vi "test Write Configuration File.vi"(8 "error in (no error)":errorcluster, 11 "TestCase in":refnum<class "Configuration Tests.lvclass">) -> (0 "error out":errorcluster, 3 "TestCase out":refnum<class "Configuration Tests.lvclass">)   [LabVIEW 2017, in "Configuration Tests.lvclass"]
uses:
  Configuration Tests.lvclass
  Configuration/Public/Controls/DSF Engine Framework Configuration.ctl
  Configuration/Public/Controls/DSF Engine Plugin Configuration.ctl
  Configuration/Public/Controls/DSF Timing Info.ctl
  Configuration/Public/Controls/DSF Engine Transfer Group Configuration.ctl
  Configuration/Public/Controls/DSF Direction.ctl
  Configuration/Public/Controls/DSF Engine Transfer Configuration.ctl
  Configuration/Public/Controls/DSF Byte Order.ctl
  Configuration/Public/Controls/DSF Engine Channel Configuration.ctl
  Configuration/Public/Controls/DSF Data Type.ctl
  Configuration/Public/Controls/DSF Settings Info.ctl
  Configuration/Public/Controls/DSF Plugin Info.ctl
  Configuration/Public/Controls/DSF Group Info.ctl
  Configuration/Public/Controls/DSF Transfer Info.ctl
  Configuration/Public/Controls/DSF Channel Info.ctl
  Configuration/Public/Write Item/Write Settings.vi
  Configuration/Public/Write Item/Write Channel.vi
  Configuration/Public/Write Item/Write Transfer.vi
  Configuration/Public/Write Item/Write Group.vi
  Configuration/Public/Write Item/Write Plugin.vi
  <vilib>/addons/_JKI Toolkits/VI Tester/TestCase.llb/TestCase.lvclass
  Configuration/Configuration Session.lvclass
  DSF Core.lvlib
  C:/Program Files (x86)/National Instruments/LabVIEW 2017/vi.lib/addons/_JKI Toolkits/VI Tester/TestCase.llb/TestCase.lvclass
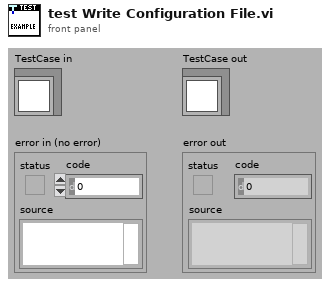
[diagram p1: front panel]
types:
  T1 = typedef "DSF Core.lvlib/DSF Settings Info.ctl" = cluster{"key":string, "value":string}[]
  T2 = typedef "DSF Core.lvlib/DSF Plugin Info.ctl" = cluster{"type":string, "timing":T3, "group ids":string[], "settings id":string, "thread count":i32}
  T3 = typedef "DSF Core.lvlib/DSF Timing Info.ctl" = cluster{"priority":u64, "decimation":u64, "offset":u64}
  T4 = typedef "DSF Core.lvlib/DSF Group Info.ctl" = cluster{"direction":T5, "timing":T3, "transfer ids":string[], "settings id":string}
  T5 = typedef "DSF Core.lvlib/DSF Direction.ctl" = enum8{"Tx", "Rx"}
  T6 = typedef "DSF Core.lvlib/DSF Transfer Info.ctl" = cluster{"byte order":T7, "channel ids":string[], "settings id":string}
  T7 = typedef "DSF Core.lvlib/DSF Byte Order.ctl" = enum8{"big-endian", "little-endian"}
  T8 = typedef "DSF Core.lvlib/DSF Channel Info.ctl" = cluster{"count":u64, "buffer offset":u64, "data type":T9, "settings id":string}
  T9 = typedef "DSF Core.lvlib/DSF Data Type.ctl" = enum8{"Bool", "SGL", "DBL", "I8", "I16", "I32", "I64", "U8", "U16", "U32", "U64"}
  T10 = typedef "DSF Core.lvlib/DSF Engine Framework Configuration.ctl" = cluster{"Plugins":T11[]}
  T11 = typedef "DSF Core.lvlib/DSF Engine Plugin Configuration.ctl" = cluster{"name":string, "class":string, "cycle timing":T3, "Transfer Groups":T12[], "settings":T1, "thread count":i32}
  T12 = typedef "DSF Core.lvlib/DSF Engine Transfer Group Configuration.ctl" = cluster{"name":string, "direction":T5, "cycle timing":T3, "Transfers":T13[], "settings":T1}
  T13 = typedef "DSF Core.lvlib/DSF Engine Transfer Configuration.ctl" = cluster{"name":string, "byte order":T7, "channel configurations":T14[], "settings":T1}
  T14 = typedef "DSF Core.lvlib/DSF Engine Channel Configuration.ctl" = cluster{"engine offset":u64, "name":string, "data type":T9, "count":u64, "buffer offset":u64}
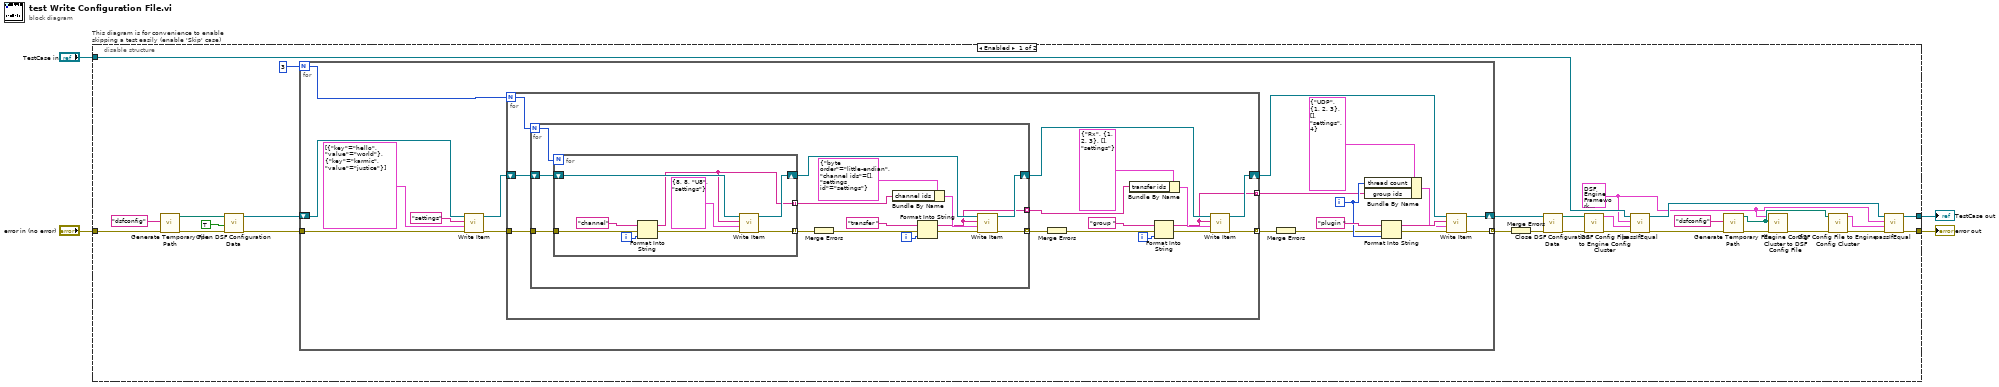
[diagram p0: block diagram]
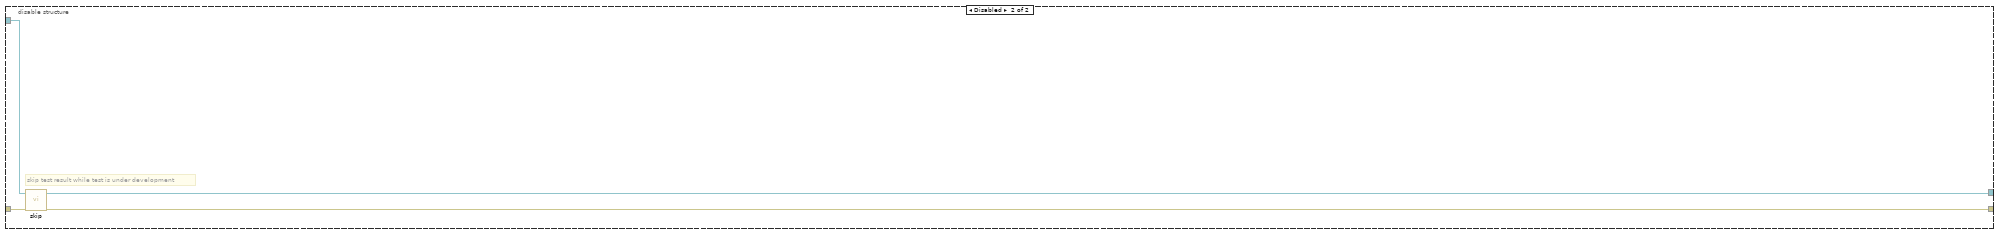
[diagram p2: hidden frame]
diagram:
  n1 = disable-structure "This diagram is for convenience to enable skipping a test easily (enable 'Skip' case)" shown="Enabled" {
    disable-tunnel: "TestCase in" -> [w18 w93]
    disable-tunnel: [w10 w91] -> w1
    disable-tunnel: [w12 w92] -> w3
    disable-tunnel: "error in (no error)" -> [w31 w90]
    frame Enabled {
      w5 = T10 {"Plugins"=[{"name"="plugin 0", "class"="UDP", "cycle timing"={"priority"=1, "decimation"=2, "offset"=3}, "Transfer Groups"=[{"name"="group 0", "direction"=enum."Rx", "cycle timing"={"priority"=1, "decimation"=2, "offset"=3}, "Transfers"=[{"name"="transfer 0", "byte order"=enum."little-endian", "channel configurations"=[{"engine offset"=0, "name"="channel0", "data type"=enum."U8", "count"=8, "buffer offset"=8}, {"engine offset"=0, "name"="channel1", "data type"=enum."U8", "count"=8, "buffer offset"=8}, {"engine offset"=0, "name"="channel2", "data type"=enum."U8", "count"=8, "buffer offset"=8}], "settings"=[{"key"="hello", "value"="world"}, {"key"="karmic", "value"="justice"}]}, {"name"="transfer 1", "byte order"=enum."little-endian", "channel configurations"=[{"engine offset"=0, "name"="channel0", "data type"=enum."U8", "count"=8, "buffer offset"=8}, {"engine offset"=0, "name"="channel1", "data type"=enum."U8", "count"=8, "buffer offset"=8}, {"engine offset"=0, "name"="channel2", "data type"=enum."U8", "count"=8, "buffer offset"=8}], "settings"=[{"key"="hello", "value"="world"}, {"key"="karmic", "value"="justice"}]}, {"name"="transfer 2", "byte order"=enum."little-endian", "channel configurations"=[{"engine offset"=0, "name"="channel0", "data type"=enum."U8", "count"=8, "buffer offset"=8}, {"engine offset"=0, "name"="channel1", "data type"=enum."U8", "count"=8, "buffer offset"=8}, {"engine offset"=0, "name"="channel2", "data type"=enum."U8", "count"=8, "buffer offset"=8}], "settings"=[{"key"="hello", "value"="world"}, {"key"="karmic", "value"="justice"}]}], "settings"=[{"key"="hello", "value"="world"}, {"key"="karmic", "value"="justice"}]}, {"name"="group 1", "direction"=enum."Rx", "cycle timing"={"priority"=1, "decimation"=2, "offset"=3}, "Transfers"=[{"name"="transfer 0", "byte order"=enum."little-endian", "channel configurations"=[{"engine offset"=0, "name"="channel0", "data type"=enum."U8", "count"=8, "buffer offset"=8}, {"engine offset"=0, "name"="channel1", "data type"=enum."U8", "count"=8, "buffer offset"=8}, {"engine offset"=0, "name"="channel2", "data type"=enum."U8", "count"=8, "buffer offset"=8}], "settings"=[{"key"="hello", "value"="world"}, {"key"="karmic", "value"="justice"}]}, {"name"="transfer 1", "byte order"=enum."little-endian", "channel configurations"=[{"engine offset"=0, "name"="channel0", "data type"=enum."U8", "count"=8, "buffer offset"=8}, {"engine offset"=0, "name"="channel1", "data type"=enum."U8", "count"=8, "buffer offset"=8}, {"engine offset"=0, "name"="channel2", "data type"=enum."U8", "count"=8, "buffer offset"=8}], "settings"=[{"key"="hello", "value"="world"}, {"key"="karmic", "value"="justice"}]}, {"name"="transfer 2", "byte order"=enum."little-endian", "channel configurations"=[{"engine offset"=0, "name"="channel0", "data type"=enum."U8", "count"=8, "buffer offset"=8}, {"engine offset"=0, "name"="channel1", "data type"=enum."U8", "count"=8, "buffer offset"=8}, {"engine offset"=0, "name"="channel2", "data type"=enum."U8", "count"=8, "buffer offset"=8}], "settings"=[{"key"="hello", "value"="world"}, {"key"="karmic", "value"="justice"}]}], "settings"=[{"key"="hello", "value"="world"}, {"key"="karmic", "value"="justice"}]}, {"name"="group 2", "direction"=enum."Rx", "cycle timing"={"priority"=1, "decimation"=2, "offset"=3}, "Transfers"=[{"name"="transfer 0", "byte order"=enum."little-endian", "channel configurations"=[{"engine offset"=0, "name"="channel0", "data type"=enum."U8", "count"=8, "buffer offset"=8}, {"engine offset"=0, "name"="channel1", "data type"=enum."U8", "count"=8, "buffer offset"=8}, {"engine offset"=0, "name"="channel2", "data type"=enum."U8", "count"=8, "buffer offset"=8}], "settings"=[{"key"="hello", "value"="world"}, {"key"="karmic", "value"="justice"}]}, {"name"="transfer 1", "byte order"=enum."little-endian", "channel configurations"=[{"engine offset"=0, "name"="channel0", "data type"=enum."U8", "count"=8, "buffer offset"=8}, {"engine offset"=0, "name"="channel1", "data type"=enum."U8", "count"=8, "buffer offset"=8}, {"engine offset"=0, "name"="channel2", "data type"=enum."U8", "count"=8, "buffer offset"=8}], "settings"=[{"key"="hello", "value"="world"}, {"key"="karmic", "value"="justice"}]}, {"name"="transfer 2", "byte order"=enum."little-endian", "channel configurations"=[{"engine offset"=0, "name"="channel0", "data type"=enum."U8", "count"=8, "buffer offset"=8}, {"engine offset"=0, "name"="channel1", "data type"=enum."U8", "count"=8, "buffer offset"=8}, {"engine offset"=0, "name"="channel2", "data type"=enum."U8", "count"=8, "buffer offset"=8}], "settings"=[{"key"="hello", "value"="world"}, {"key"="karmic", "value"="justice"}]}], "settings"=[{"key"="hello", "value"="world"}, {"key"="karmic", "value"="justice"}]}], "settings"=[{"key"="hello", "value"="world"}, {"key"="karmic", "value"="justice"}], "thread count"=0}, {"name"="plugin 1", "class"="UDP", "cycle timing"={"priority"=1, "decimation"=2, "offset"=3}, "Transfer Groups"=[{"name"="group 0", "direction"=enum."Rx", "cycle timing"={"priority"=1, "decimation"=2, "offset"=3}, "Transfers"=[{"name"="transfer 0", "byte order"=enum."little-endian", "channel configurations"=[{"engine offset"=0, "name"="channel0", "data type"=enum."U8", "count"=8, "buffer offset"=8}, {"engine offset"=0, "name"="channel1", "data type"=enum."U8", "count"=8, "buffer offset"=8}, {"engine offset"=0, "name"="channel2", "data type"=enum."U8", "count"=8, "buffer offset"=8}], "settings"=[{"key"="hello", "value"="world"}, {"key"="karmic", "value"="justice"}]}, {"name"="transfer 1", "byte order"=enum."little-endian", "channel configurations"=[{"engine offset"=0, "name"="channel0", "data type"=enum."U8", "count"=8, "buffer offset"=8}, {"engine offset"=0, "name"="channel1", "data type"=enum."U8", "count"=8, "buffer offset"=8}, {"engine offset"=0, "name"="channel2", "data type"=enum."U8", "count"=8, "buffer offset"=8}], "settings"=[{"key"="hello", "value"="world"}, {"key"="karmic", "value"="justice"}]}, {"name"="transfer 2", "byte order"=enum."little-endian", "channel configurations"=[{"engine offset"=0, "name"="channel0", "data type"=enum."U8", "count"=8, "buffer offset"=8}, {"engine offset"=0, "name"="channel1", "data type"=enum."U8", "count"=8, "buffer offset"=8}, {"engine offset"=0, "name"="channel2", "data type"=enum."U8", "count"=8, "buffer offset"=8}], "settings"=[{"key"="hello", "value"="world"}, {"key"="karmic", "value"="justice"}]}], "settings"=[{"key"="hello", "value"="world"}, {"key"="karmic", "value"="justice"}]}, {"name"="group 1", "direction"=enum."Rx", "cycle timing"={"priority"=1, "decimation"=2, "offset"=3}, "Transfers"=[{"name"="transfer 0", "byte order"=enum."little-endian", "channel configurations"=[{"engine offset"=0, "name"="channel0", "data type"=enum."U8", "count"=8, "buffer offset"=8}, {"engine offset"=0, "name"="channel1", "data type"=enum."U8", "count"=8, "buffer offset"=8}, {"engine offset"=0, "name"="channel2", "data type"=enum."U8", "count"=8, "buffer offset"=8}], "settings"=[{"key"="hello", "value"="world"}, {"key"="karmic", "value"="justice"}]}, {"name"="transfer 1", "byte order"=enum."little-endian", "channel configurations"=[{"engine offset"=0, "name"="channel0", "data type"=enum."U8", "count"=8, "buffer offset"=8}, {"engine offset"=0, "name"="channel1", "data type"=enum."U8", "count"=8, "buffer offset"=8}, {"engine offset"=0, "name"="channel2", "data type"=enum."U8", "count"=8, "buffer offset"=8}], "settings"=[{"key"="hello", "value"="world"}, {"key"="karmic", "value"="justice"}]}, {"name"="transfer 2", "byte order"=enum."little-endian", "channel configurations"=[{"engine offset"=0, "name"="channel0", "data type"=enum."U8", "count"=8, "buffer offset"=8}, {"engine offset"=0, "name"="channel1", "data type"=enum."U8", "count"=8, "buffer offset"=8}, {"engine offset"=0, "name"="channel2", "data type"=enum."U8", "count"=8, "buffer offset"=8}], "settings"=[{"key"="hello", "value"="world"}, {"key"="karmic", "value"="justice"}]}], "settings"=[{"key"="hello", "value"="world"}, {"key"="karmic", "value"="justice"}]}, {"name"="group 2", "direction"=enum."Rx", "cycle timing"={"priority"=1, "decimation"=2, "offset"=3}, "Transfers"=[{"name"="transfer 0", "byte order"=enum."little-endian", "channel configurations"=[{"engine offset"=0, "name"="channel0", "data type"=enum."U8", "count"=8, "buffer offset"=8}, {"engine offset"=0, "name"="channel1", "data type"=enum."U8", "count"=8, "buffer offset"=8}, {"engine offset"=0, "name"="channel2", "data type"=enum."U8", "count"=8, "buffer offset"=8}], "settings"=[{"key"="hello", "value"="world"}, {"key"="karmic", "value"="justice"}]}, {"name"="transfer 1", "byte order"=enum."little-endian", "channel configurations"=[{"engine offset"=0, "name"="channel0", "data type"=enum."U8", "count"=8, "buffer offset"=8}, {"engine offset"=0, "name"="channel1", "data type"=enum."U8", "count"=8, "buffer offset"=8}, {"engine offset"=0, "name"="channel2", "data type"=enum."U8", "count"=8, "buffer offset"=8}], "settings"=[{"key"="hello", "value"="world"}, {"key"="karmic", "value"="justice"}]}, {"name"="transfer 2", "byte order"=enum."little-endian", "channel configurations"=[{"engine offset"=0, "name"="channel0", "data type"=enum."U8", "count"=8, "buffer offset"=8}, {"engine offset"=0, "name"="channel1", "data type"=enum."U8", "count"=8, "buffer offset"=8}, {"engine offset"=0, "name"="channel2", "data type"=enum."U8", "count"=8, "buffer offset"=8}], "settings"=[{"key"="hello", "value"="world"}, {"key"="karmic", "value"="justice"}]}], "settings"=[{"key"="hello", "value"="world"}, {"key"="karmic", "value"="justice"}]}], "settings"=[{"key"="hello", "value"="world"}, {"key"="karmic", "value"="justice"}], "thread count"=1}, {"name"="plugin 2", "class"="UDP", "cycle timing"={"priority"=1, "decimation"=2, "offset"=3}, "Transfer Groups"=[{"name"="group 0", "direction"=enum."Rx", "cycle timing"={"priority"=1, "decimation"=2, "offset"=3}, "Transfers"=[{"name"="transfer 0", "byte order"=enum."little-endian", "channel configurations"=[{"engine offset"=0, "name"="channel0", "data type"=enum."U8", "count"=8, "buffer offset"=8}, {"engine offset"=0, "name"="channel1", "data type"=enum."U8", "count"=8, "buffer offset"=8}, {"engine offset"=0, "name"="channel2", "data type"=enum."U8", "count"=8, "buffer offset"=8}], "settings"=[{"key"="hello", "value"="world"}, {"key"="karmic", "value"="justice"}]}, {"name"="transfer 1", "byte order"=enum."little-endian", "channel configurations"=[{"engine offset"=0, "name"="channel0", "data type"=enum."U8", "count"=8, "buffer offset"=8}, {"engine offset"=0, "name"="channel1", "data type"=enum."U8", "count"=8, "buffer offset"=8}, {"engine offset"=0, "name"="channel2", "data type"=enum."U8", "count"=8, "buffer offset"=8}], "settings"=[{"key"="hello", "value"="world"}, {"key"="karmic", "value"="justice"}]}, {"name"="transfer 2", "byte order"=enum."little-endian", "channel configurations"=[{"engine offset"=0, "name"="channel0", "data type"=enum."U8", "count"=8, "buffer offset"=8}, {"engine offset"=0, "name"="channel1", "data type"=enum."U8", "count"=8, "buffer offset"=8}, {"engine offset"=0, "name"="channel2", "data type"=enum."U8", "count"=8, "buffer offset"=8}], "settings"=[{"key"="hello", "value"="world"}, {"key"="karmic", "value"="justice"}]}], "settings"=[{"key"="hello", "value"="world"}, {"key"="karmic", "value"="justice"}]}, {"name"="group 1", "direction"=enum."Rx", "cycle timing"={"priority"=1, "decimation"=2, "offset"=3}, "Transfers"=[{"name"="transfer 0", "byte order"=enum."little-endian", "channel configurations"=[{"engine offset"=0, "name"="channel0", "data type"=enum."U8", "count"=8, "buffer offset"=8}, {"engine offset"=0, "name"="channel1", "data type"=enum."U8", "count"=8, "buffer offset"=8}, {"engine offset"=0, "name"="channel2", "data type"=enum."U8", "count"=8, "buffer offset"=8}], "settings"=[{"key"="hello", "value"="world"}, {"key"="karmic", "value"="justice"}]}, {"name"="transfer 1", "byte order"=enum."little-endian", "channel configurations"=[{"engine offset"=0, "name"="channel0", "data type"=enum."U8", "count"=8, "buffer offset"=8}, {"engine offset"=0, "name"="channel1", "data type"=enum."U8", "count"=8, "buffer offset"=8}, {"engine offset"=0, "name"="channel2", "data type"=enum."U8", "count"=8, "buffer offset"=8}], "settings"=[{"key"="hello", "value"="world"}, {"key"="karmic", "value"="justice"}]}, {"name"="transfer 2", "byte order"=enum."little-endian", "channel configurations"=[{"engine offset"=0, "name"="channel0", "data type"=enum."U8", "count"=8, "buffer offset"=8}, {"engine offset"=0, "name"="channel1", "data type"=enum."U8", "count"=8, "buffer offset"=8}, {"engine offset"=0, "name"="channel2", "data type"=enum."U8", "count"=8, "buffer offset"=8}], "settings"=[{"key"="hello", "value"="world"}, {"key"="karmic", "value"="justice"}]}], "settings"=[{"key"="hello", "value"="world"}, {"key"="karmic", "value"="justice"}]}, {"name"="group 2", "direction"=enum."Rx", "cycle timing"={"priority"=1, "decimation"=2, "offset"=3}, "Transfers"=[{"name"="transfer 0", "byte order"=enum."little-endian", "channel configurations"=[{"engine offset"=0, "name"="channel0", "data type"=enum."U8", "count"=8, "buffer offset"=8}, {"engine offset"=0, "name"="channel1", "data type"=enum."U8", "count"=8, "buffer offset"=8}, {"engine offset"=0, "name"="channel2", "data type"=enum."U8", "count"=8, "buffer offset"=8}], "settings"=[{"key"="hello", "value"="world"}, {"key"="karmic", "value"="justice"}]}, {"name"="transfer 1", "byte order"=enum."little-endian", "channel configurations"=[{"engine offset"=0, "name"="channel0", "data type"=enum."U8", "count"=8, "buffer offset"=8}, {"engine offset"=0, "name"="channel1", "data type"=enum."U8", "count"=8, "buffer offset"=8}, {"engine offset"=0, "name"="channel2", "data type"=enum."U8", "count"=8, "buffer offset"=8}], "settings"=[{"key"="hello", "value"="world"}, {"key"="karmic", "value"="justice"}]}, {"name"="transfer 2", "byte order"=enum."little-endian", "channel configurations"=[{"engine offset"=0, "name"="channel0", "data type"=enum."U8", "count"=8, "buffer offset"=8}, {"engine offset"=0, "name"="channel1", "data type"=enum."U8", "count"=8, "buffer offset"=8}, {"engine offset"=0, "name"="channel2", "data type"=enum."U8", "count"=8, "buffer offset"=8}], "settings"=[{"key"="hello", "value"="world"}, {"key"="karmic", "value"="justice"}]}], "settings"=[{"key"="hello", "value"="world"}, {"key"="karmic", "value"="justice"}]}], "settings"=[{"key"="hello", "value"="world"}, {"key"="karmic", "value"="justice"}], "thread count"=2}]} ("framework configuration out")
      n2 = call <vilib>:"Generate Temporary File Path.vi"("error in (no error)"=w31, "Temporary File Extension (tmp)"="dsfconfig") -> ("error out"=w29:errorcluster, "Unique Temporary File Path"=w28:path)  [unwired: 8 in]
      n3 = call "Open DSF Configuration Data.vi"("error in (no error)"=w29, "replace if found? (F)"=TRUE, "dsf configuration file path"=w28) -> ("error out"=w26:errorcluster, "Configuration Session"=w22:refnum<class "Configuration Session.lvclass">)  [unwired: 4 in, 3 out]
      n4 = for {
        N: 3 -> [w34]
        tunnel: w26 -> [w43]
        tunnel: [w37] -> w23 mode=indexing
        shift-right: [w33] -> w21
        shift-left: w22 -> [w32]
        i -> [w46]
        n5 = call-poly "Write Item.vi"("error in (no error)"=w43, "settings values"=T1 [{"key"="hello", "value"="world"}, {"key"="karmic", "value"="justice"}], "id"="settings", "Configuration Session in"=w32) -> ("error out"=w36:errorcluster, "Configuration Session out"=w41:refnum<class "Configuration Session.lvclass">)  [unwired: 5 in, 1 out]
        n6 = for {
          N: w34 -> [w51]
          tunnel: [w56] -> w42 mode=indexing
          shift-right: [w59] -> w40
          shift-left: w41 -> [w61]
          tunnel: w36 -> [w55]
          tunnel: [w52] -> w35 mode=indexing
          i -> [w63]
          n7 = for {
            N: w51 -> [w66]
            tunnel: [w72] -> w62 mode=indexing
            shift-right: [w75] -> w60
            shift-left: w61 -> [w78]
            tunnel: w55 -> [w71]
            tunnel: [w67] -> w53 mode=indexing
            i -> [w77]
            n8 = for {
              N: w66 -> [_]
              tunnel: [w86] -> w79 mode=indexing
              shift-right: [w83] -> w76
              shift-left: w78 -> [w89]
              tunnel: w71 -> [w85]
              tunnel: [w82] -> w68 mode=indexing
              i -> [w81]
              n9 = Format Into String(initial string="channel" ("id"), error in=w85, w81) -> (resulting string=w82:string, error out=w84:errorcluster)  [unwired: 1 in]
              n10 = call-poly "Write Item.vi"("error in (no error)"=w84, "channel values"=T8 {"count"=8, "buffer offset"=8, "data type"=enum."U8", "settings id"="settings"}, "id"=w82, "Configuration Session in"=w89) -> ("error out"=w86:errorcluster, "Configuration Session out"=w83:refnum<class "Configuration Session.lvclass">)  [unwired: 5 in, 1 out]
            }
            n11 = Merge Errors(w79) -> (w74:errorcluster)
            n12 = Bundle By Name(cluster=T6 {"byte order"=enum."little-endian", "channel ids"=[], "settings id"="settings"} ("transfer values"), "channel ids"=w68) -> (w69:T6)
            n13 = Format Into String(initial string="transfer ", error in=w74, w77) -> (resulting string=w67:string, error out=w73:errorcluster)  [unwired: 1 in]
            n14 = call-poly "Write Item.vi"("error in (no error)"=w73, "transfer values"=w69, "id"=w67, "Configuration Session in"=w76) -> ("error out"=w72:errorcluster, "Configuration Session out"=w75:refnum<class "Configuration Session.lvclass">)  [unwired: 5 in, 1 out]
          }
          n15 = Merge Errors(w62) -> (w58:errorcluster)
          n16 = Bundle By Name(cluster=T4 {"direction"=enum."Rx", "timing"={"priority"=1, "decimation"=2, "offset"=3}, "transfer ids"=[], "settings id"="settings"} ("group values"), "transfer ids"=w53) -> (w54:T4)
          n17 = Format Into String(initial string="group ", error in=w58, w63) -> (resulting string=w52:string, error out=w57:errorcluster)  [unwired: 1 in]
          n18 = call-poly "Write Item.vi"("error in (no error)"=w57, "group values"=w54, "id"=w52, "Configuration Session in"=w60) -> ("error out"=w56:errorcluster, "Configuration Session out"=w59:refnum<class "Configuration Session.lvclass">)  [unwired: 5 in, 1 out]
        }
        n19 = Merge Errors(w42) -> (w39:errorcluster)
        n20 = Bundle By Name(cluster=T2 {"type"="UDP", "timing"={"priority"=1, "decimation"=2, "offset"=3}, "group ids"=[], "settings id"="settings", "thread count"=4} ("plugin values"), "thread count"=w46, "group ids"=w35) -> (w47:T2)
        n21 = Format Into String(initial string="plugin ", error in=w39, w46) -> (resulting string=w49:string, error out=w38:errorcluster)  [unwired: 1 in]
        n22 = call-poly "Write Item.vi"("error in (no error)"=w38, "plugin values"=w47, "id"=w49, "Configuration Session in"=w40) -> ("error out"=w37:errorcluster, "Configuration Session out"=w33:refnum<class "Configuration Session.lvclass">)  [unwired: 5 in, 1 out]
      }
      n23 = Merge Errors(w23) -> (w25:errorcluster)
      n24 = call "Close DSF Configuration Data.vi"("error in (no error)"=w25, "Configuration Session"=w21) -> ("error out"=w20:errorcluster, "file path"=w13:path)  [unwired: 8 in]
      n25 = call "DSF Config File to Engine Config Cluster.vi"("error in (no error)"=w20, "dsf configuration file path"=w13) -> ("error out"=w19:errorcluster, "framework configuration out"=w17:T10)  [unwired: 8 in]
      n26 = call-dynamic "passIfEqual.vi"("error in (no error)"=w19, "y"=w17, "x"=w5, "TestCase in"=w18) -> ("error out"=w15:errorcluster, "TestCase out"=w11:refnum<class "Configuration Tests.lvclass">)  [unwired: 6 in]
      n27 = call <vilib>:"Generate Temporary File Path.vi"("error in (no error)"=w15, "Temporary File Extension (tmp)"="dsfconfig") -> ("error out"=w14:errorcluster, "Unique Temporary File Path"=w7:path)  [unwired: 8 in]
      n28 = call "Engine Config Cluster to DSF Config File.vi"("error in (no error)"=w14, "dsf configuration file path"=w7, "framework configuration"=w5) -> ("error out"=w9:errorcluster)  [unwired: 8 in]
      n29 = call "DSF Config File to Engine Config Cluster.vi"("error in (no error)"=w9, "dsf configuration file path"=w7) -> ("error out"=w8:errorcluster, "framework configuration out"=w6:T10)  [unwired: 8 in]
      n30 = call-dynamic "passIfEqual.vi"("error in (no error)"=w8, "y"=w6, "x"=w5, "TestCase in"=w11) -> ("error out"=w12:errorcluster, "TestCase out"=w10:refnum<class "Configuration Tests.lvclass">)  [unwired: 6 in]
    }
    frame Disabled {
      # "skip test result while test is under development"
      n31 = call <vilib>:"skip.vi"("error in (no error)"=w90, "TestCase in"=w93) -> ("error out"=w92:errorcluster, "TestCase out"=w91:refnum<class "Configuration Tests.lvclass">)  [unwired: 8 in]
    }
  }
  "error out" <- w3
  "TestCase out" <- w1
